vi "Write OCP_Mode.vi"(8 "error in":errorcluster, 10 "OCP Mode":T1, 11 "57XX in":refnum<class "57XX.lvclass">) -> (0 "error out":errorcluster, 3 "57XX out":refnum<class "57XX.lvclass">)   [LabVIEW 2019, in "57XX.lvlib" / "57XX.lvclass"]
uses:
  Library/57XX.lvclass
  C:/Users/Public/Documents/Development/builds/Engine/Monitored Actor.lvlibp/Monitored Actor/Monitored Actor/Monitored Actor.lvclass
  builds/Instruments/PowerSupply.lvlibp/Custom Controls/OCP Mode.ctl
  builds/Engine/Monitored Actor.lvlibp/Monitored Actor/Monitored Actor/Read Actor Label.vi
  builds/Instruments/PowerSupply.lvlibp/Library/PowerSupply.lvclass
  <vilib>/ErrorRing/Error Ring.xnode
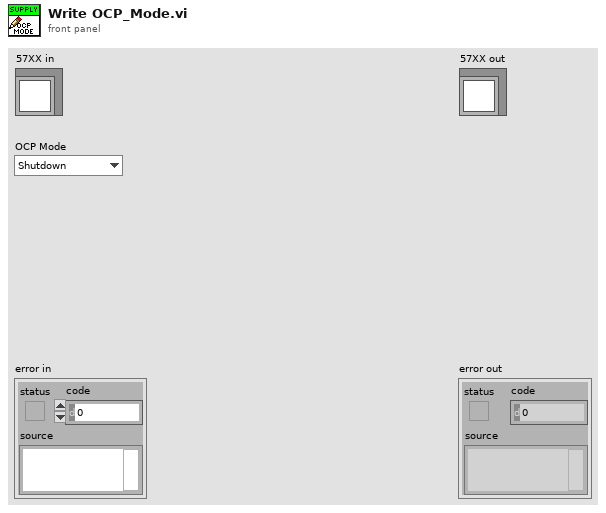
[diagram p1: front panel]
types:
  T1 = typedef "PowerSupply.lvlibp/PowerSupply.lvclass/OCP Mode.ctl" = enum16{"Shutdown", "Foldback"}
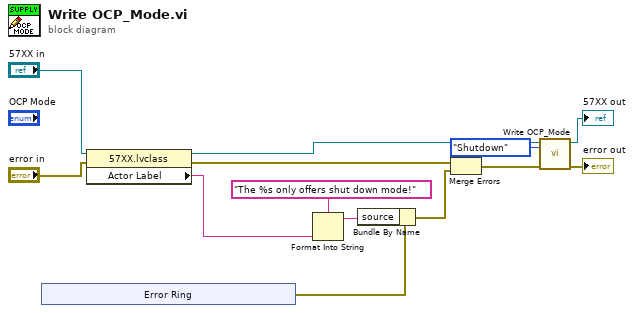
[diagram p0: block diagram]
diagram:
  n1 = xnode "Error Ring"() -> ("error out"=w7:errorcluster)
  n2 = property class="57XX.lvclass"(reference="57XX in", error in="error in") -> (reference out=w3:refnum<class "57XX.lvclass">, error out=w6:errorcluster, "Actor Label"=w10:string)
  n3 = Format Into String(format string="The %s only offers shut down mode!", w10) -> (resulting string=w8:string)  [unwired: 2 in, 1 out]
  n4 = Bundle By Name(cluster=w7, "source"=w8) -> (w9:errorcluster)
  n5 = Merge Errors(w6, w9) -> (w4:errorcluster)
  n6 = call-parent "Write OCP_Mode.vi"("error in"=w4, "OCP Mode"=OCP_Mode."Shutdown", "PowerSupply in"=w3) -> ("error out"=→"error out":errorcluster, "PowerSupply out"=→"57XX out":refnum<class "57XX.lvclass">)  [unwired: 7 in]
